vi "CreateLibIfNotPresent.vi"(8 "error in (no error)":errorcluster, 9 "DestDirectory":path, 10 "ProjectRef":refnum<vi>, 11 "VirtualFolderRef":refnum<vi>) -> (0 "error out":errorcluster, 3 "Library Refnum":refnum<vi>)   [LabVIEW 2021, in "Converter.lvlib"]
uses:
  Converter.lvlib
  Converter Reusables/Converter Reusables.lvlib
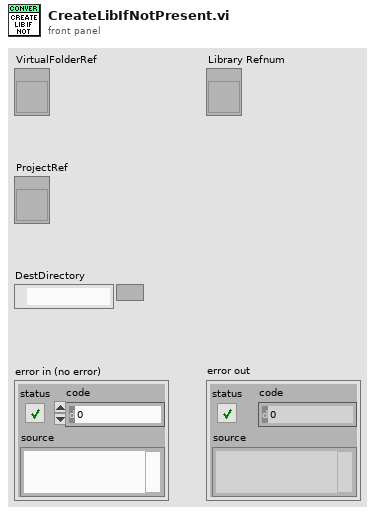
[diagram p1: front panel]
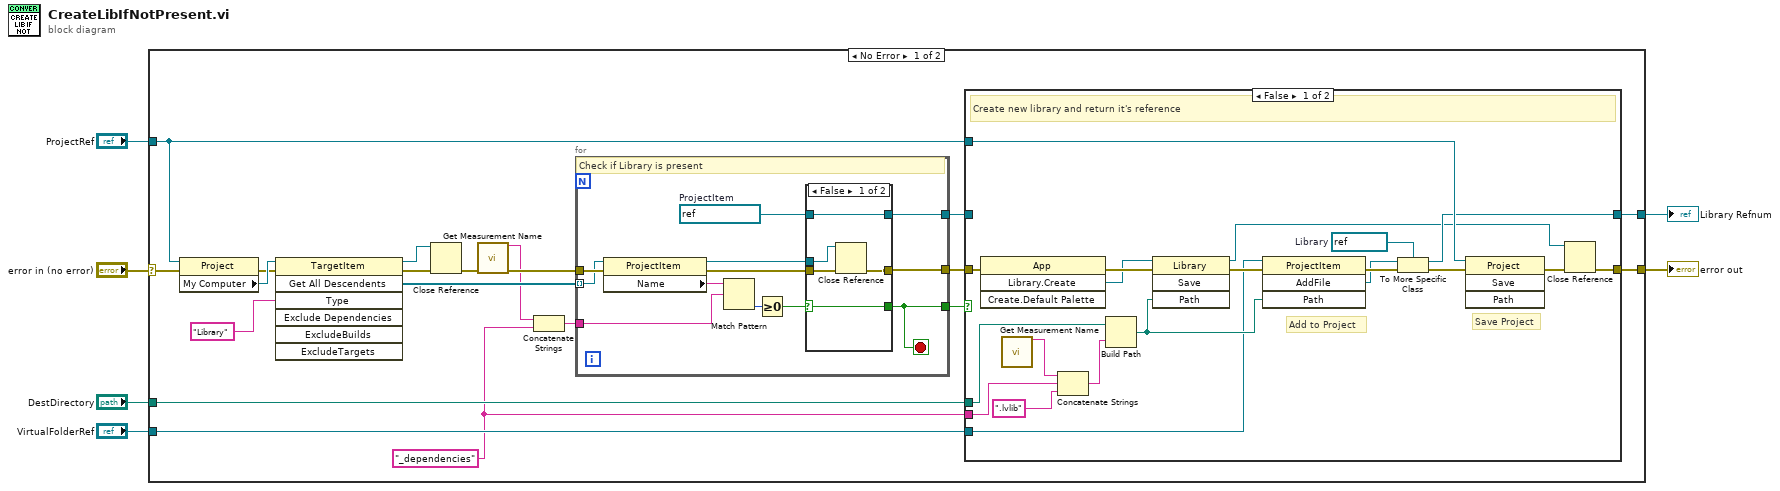
[diagram p0: block diagram]
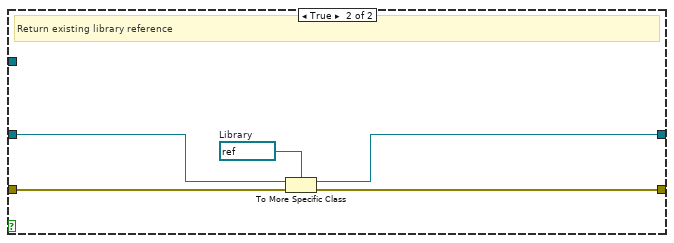
[diagram p2: hidden frame]
diagram:
  n1 = case shown="No Error" "error in (no error)" {
    selector: "error in (no error)" -> [w14 w72]
    tunnel: "DestDirectory" -> [w13 _]
    tunnel: "VirtualFolderRef" -> [w12 _]
    tunnel: "ProjectRef" -> [w11 _]
    tunnel: [w10 w72] -> w2
    tunnel: [w8 _] -> w1
    frame No Error {
      w7 = "_dependencies" ("string")
      n2 = property class="Project"(reference=w11, error in=w14) -> (error out=w22:errorcluster, "My Computer"=w26:refnum<vi>)  [unwired: 1 out]
      n3 = invoke class="TargetItem" method="Get All Descendents"(reference=w26, error in=w22, "Type"="Library") -> (reference out=w23:refnum<vi>, error out=w24:errorcluster, "All Descendents"=w21:refnum<vi>[])  [unwired: 4 in, 4 out]
      n4 = Close Reference(reference=w23, error in (no error)=w24) -> (error out=w20:errorcluster)
      n5 = call "Get Measurement Name.vi"("error in (no error)"=w20) -> ("Name Out"=w18:string, "error out"=w19:errorcluster)  [unwired: 13 in]
      n6 = Concatenate Strings(w18, w7) -> (w17:string)
      n7 = for {
        tunnel: w21 -> [w62] mode=indexing
        tunnel: w19 -> [w63]
        tunnel: [w55] -> w9
        tunnel: [w54] -> w15
        tunnel: w17 -> [w53]
        tunnel: [w52] -> w16
        stop <- w52 stop-if-true
        w58 = refnum<vi> refnum  # ProjectItem
        # "Check if Library is present"
        n8 = property class="ProjectItem"(reference=w62, error in=w63) -> (reference out=w57:refnum<vi>, error out=w56:errorcluster, "Name"=w61:string)
        n9 = Match Pattern(string=w61, regular expression=w53) -> (offset past match=w60:i32)  [unwired: 1 in, 3 out]
        n10 = Greater Or Equal To 0?(x=w60) -> (x >= 0?=w59:bool)
        n11 = case shown="False" w59 {
          selector: w59 -> [w65 w70]
          tunnel: w57 -> [w66 w71]
          tunnel: [w68 w69] -> w54
          tunnel: [w67 w71] -> w55
          tunnel: w58 -> [w67 _]
          tunnel: [w65 w70] -> w52
          tunnel: w56 -> [w64 w69]
          frame False {
            n12 = Close Reference(reference=w66, error in (no error)=w64) -> (error out=w68:errorcluster)
          }
          frame True {
          }
        }
      }
      n13 = case shown="False" w16 {
        tunnel: w15 -> [w46 w51]
        tunnel: w13 -> [w44 _]
        tunnel: w12 -> [w37 _]
        tunnel: w11 -> [w36 _]
        tunnel: [w30 w50] -> w10
        tunnel: w9 -> [_ w48]
        tunnel: [w31 w49] -> w8
        tunnel: w7 -> [w27 _]
        frame False {
          w32 = refnum<vi> refnum  # Library
          # "Save Project"
          # "Add to Project"
          # "Create new library and return it's reference"
          n14 = invoke class="App" method="Library.Create"(error in=w46) -> (error out=w45:errorcluster, "Create Library"=w41:refnum<vi>)  [unwired: 3 in, 2 out]
          n15 = call "Get Measurement Name.vi"() -> ("Name Out"=w43:string)  [unwired: 14 in, 1 out]
          n16 = Concatenate Strings(w43, w27, ".lvlib" ("string")) -> (w42:string)
          n17 = Build Path(base path=w44, name or relative path=w42) -> (appended path=w38:path)
          n18 = invoke class="Library" method="Save"(reference=w41, error in=w45, "Path"=w38) -> (reference out=w29:refnum<vi>, error out=w39:errorcluster)  [unwired: 1 in, 2 out]
          n19 = invoke class="ProjectItem" method="AddFile"(reference=w37, error in=w39, "Path"=w38) -> (error out=w40:errorcluster, "AddFile"=w33:refnum<vi>)  [unwired: 1 in, 2 out]
          n20 = To More Specific Class(target class=w32, reference=w33, error in=w40) -> (specific class reference=w31:refnum<vi>, error out=w34:errorcluster)
          n21 = invoke class="Project" method="Save"(reference=w36, error in=w34) -> (error out=w35:errorcluster)  [unwired: 2 in, 3 out]
          n22 = Close Reference(reference=w29, error in (no error)=w35) -> (error out=w30:errorcluster)
        }
        frame True {
          w47 = refnum<vi> refnum  # Library
          # "Return existing library reference"
          n23 = To More Specific Class(target class=w47, reference=w48, error in=w51) -> (specific class reference=w49:refnum<vi>, error out=w50:errorcluster)
        }
      }
    }
    frame Error {
    }
  }
  "error out" <- w2
  "Library Refnum" <- w1
